vi "深国电程序控制old.vi"(11 "槽位号":i16) -> ()   [LabVIEW 2012]
doc: "打开板卡操作，输出板卡句柄！当有多个板卡时，根据板卡索引号打开不同板卡！\n如果同时使用一块板卡的多种功能，可将输出句柄连接到不同的功能任务中。\n此VI是创建所有任务的前提！"
uses:
  P3060.dll
panel:
  out "波形图":i32[](graph)
  in  "read":bool caption="确定按钮"
  in  "LED¿ØÖÆû":bool
  in  "FPGA-Bit文件路径":path
  in  "加载程序":bool caption="确定按钮"
  in  "取消按钮":bool
  out "error out":errorcluster caption="错误输出"
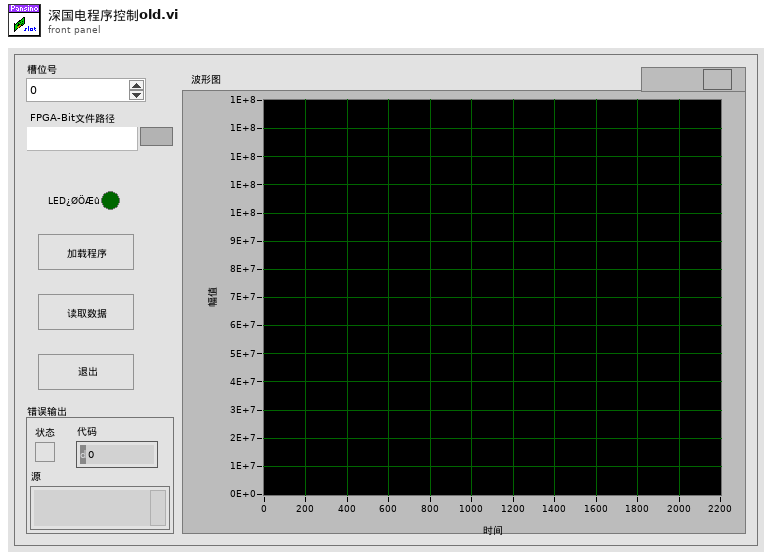
[diagram p1: front panel]
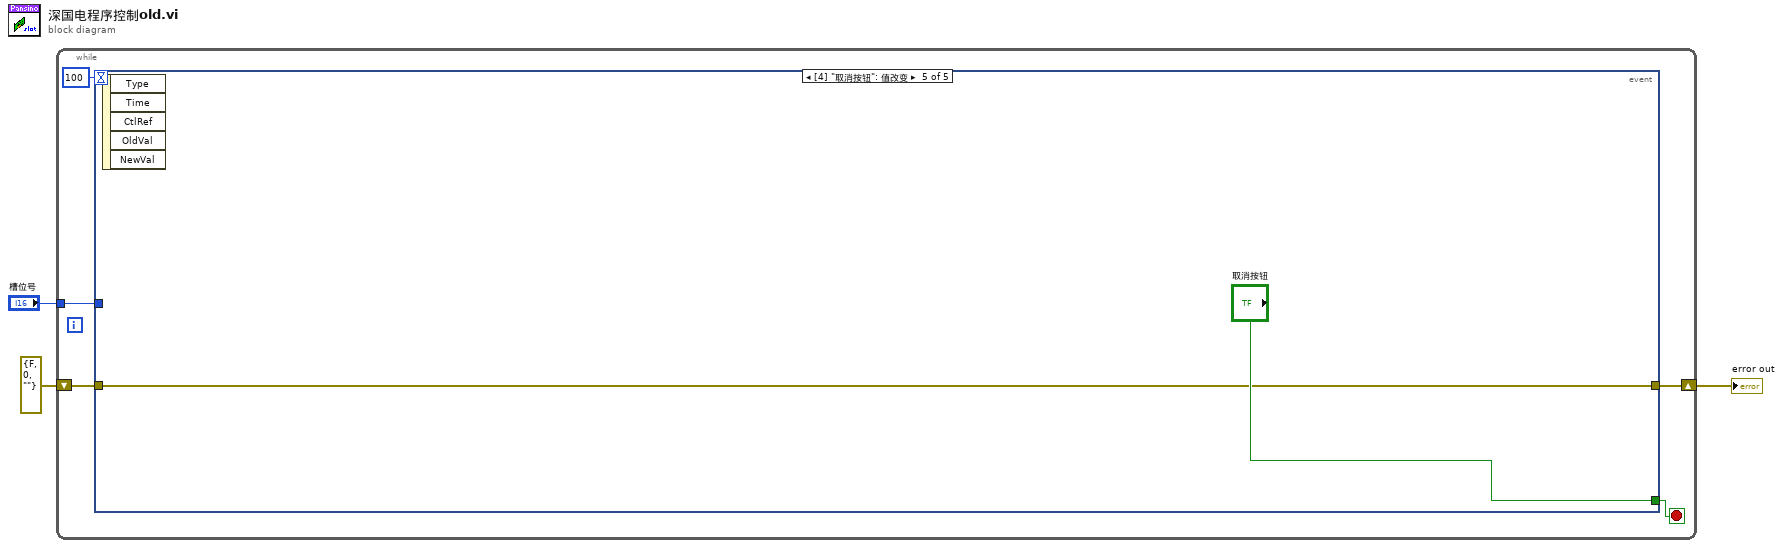
[diagram p0: block diagram]
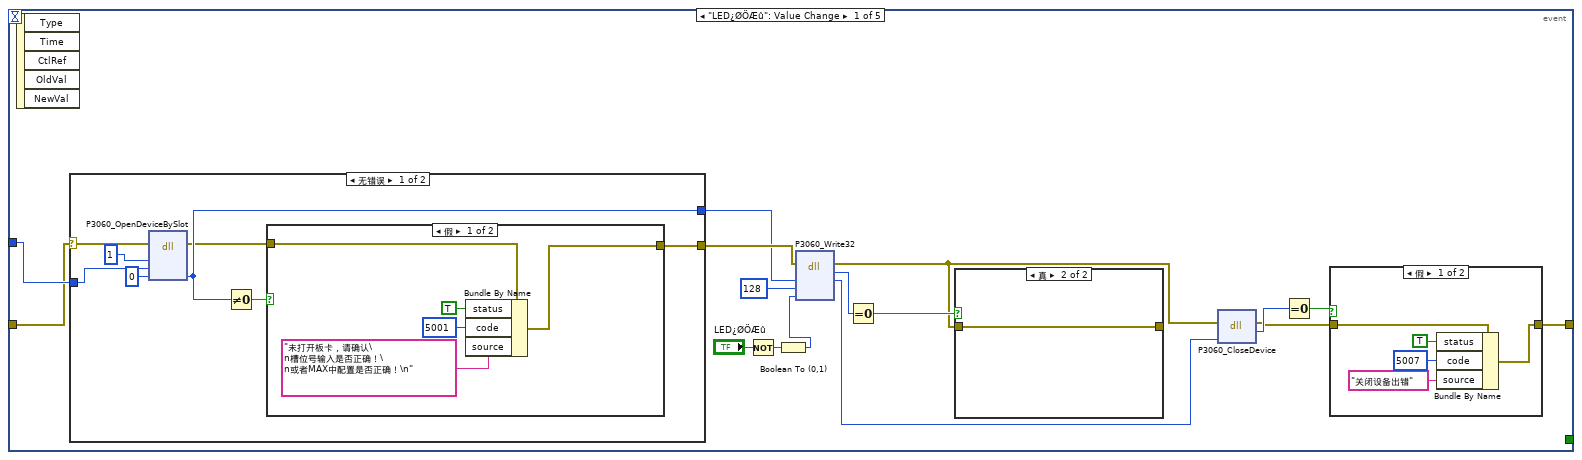
[diagram p2: hidden frame]
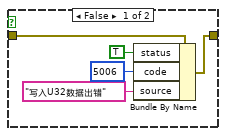
[diagram p3: hidden frame]
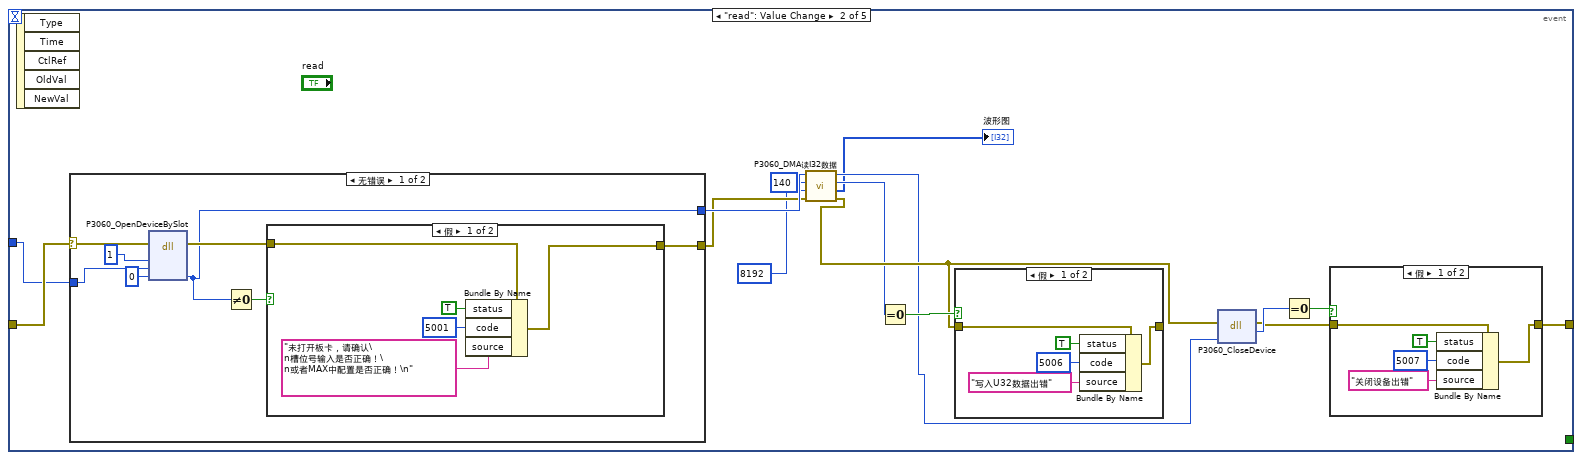
[diagram p7: hidden frame]
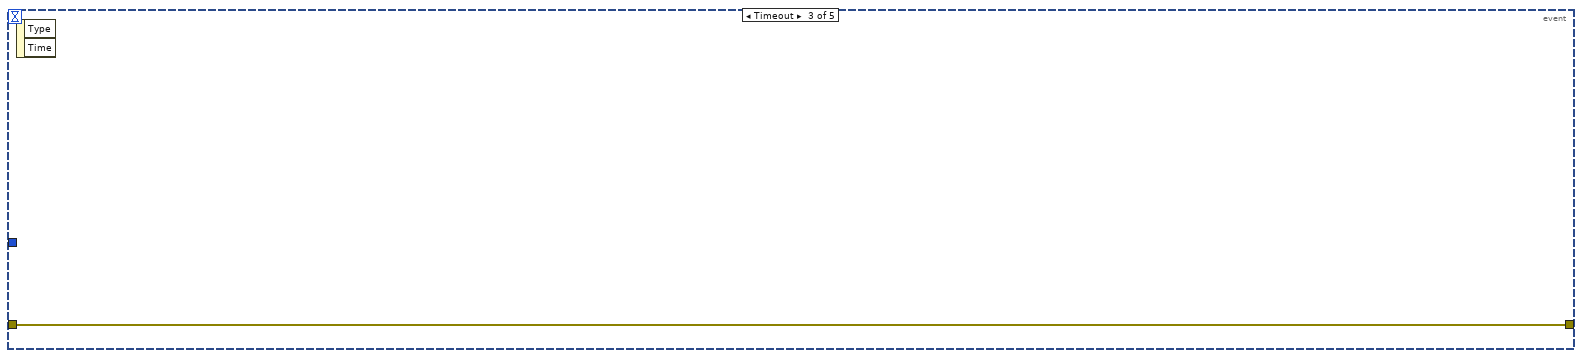
[diagram p12: hidden frame]
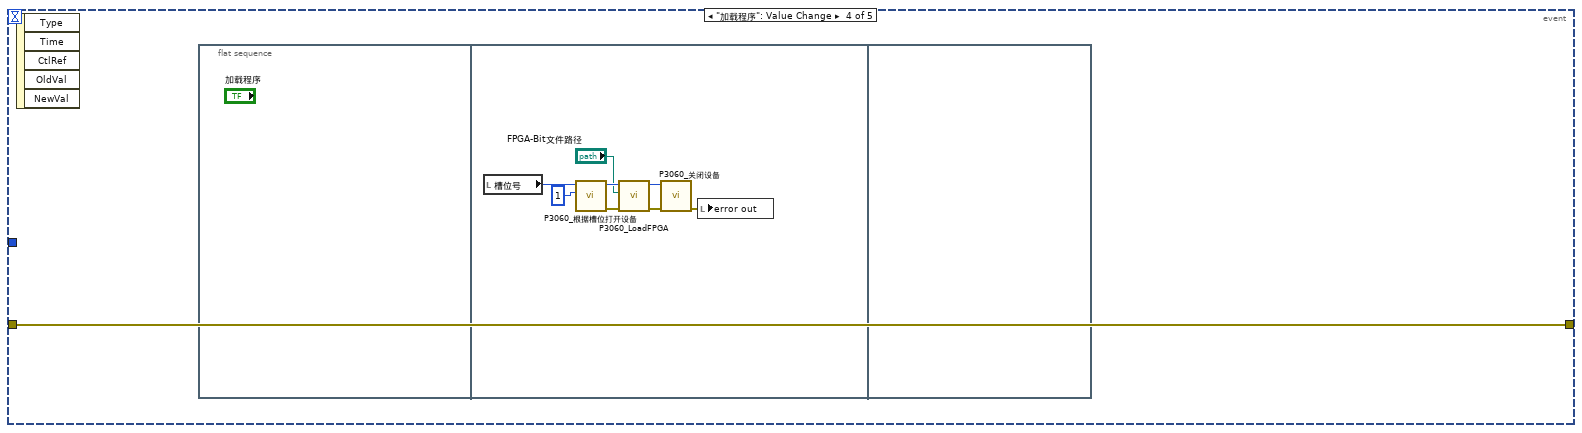
[diagram p13: hidden frame]
diagram:
  n1 = while {
    tunnel: "槽位号" -> [w8]
    shift-right: [w7] -> w1
    shift-left: errorcluster {"status"=FALSE, "code"=0, "source"=""} ("error IO") -> [w6]
    stop <- w4 stop-if-true
    n2 = event shown="[4] \"取消按钮\": 值改变" {
      selector: _ -> [_ _ _ _ _]
      dyn-events: _ -> [_ _ _ _ _]
      timeout: 100 -> [_ _ _ _ _]
      tunnel: [_ _ _ _ "取消按钮"] -> w4
      tunnel: w8 -> [w14 w52 _ _ _]
      tunnel: [w12 w62 w94 w95 w104] -> w7
      tunnel: w6 -> [w13 w61 w94 w95 w104]
      event "LED¿ØÖÆû": Value Change {
        n3 = event-data() -> ()  [unwired: 1 in, 5 out]
        n4 = case shown="无错误" w13 {
          selector: w13 -> [w44 w51]
          tunnel: [w41 w51] -> w19
          tunnel: w14 -> [w43 _]
          tunnel: [w40 _] -> w17
          frame No Error {
            n5 = dll-call lib="P3060.dll" fn="P3060_OpenDeviceBySlot"(error in=w44, "Classis"=i16 1, "槽位号"=w43, "设备句柄"=0) -> (error out=w37:errorcluster, "设备句柄"=w40:i32)  [unwired: 5 in, 1 out]
            n6 = Not Equal To 0?(x=w40) -> (x != 0?=w42:bool)
            n7 = case shown="假" w42 {
              tunnel: w37 -> [w49 w50]
              tunnel: [w45 w50] -> w41
              frame False {
                n8 = Bundle By Name(cluster=w49, "status"=TRUE, "code"=5001, "source"="未打开板卡，请确认\n槽位号输入是否正确！\n或者MAX中配置是否正确！\n") -> (w45:errorcluster)
              }
              frame True {
              }
            }
          }
          frame Error {
          }
        }
        n9 = Not(x="LED¿ØÖÆû") -> (.not. x?=w10:bool)
        n10 = Boolean To (0,1)(Boolean=w10) -> (0, 1=w11:i16)
        n11 = dll-call lib="P3060.dll" fn="P3060_Write32"(error in=w19, "hDev"=w17, "Offset"=u32 128, "data"=w11) -> (error out=w18:errorcluster, "return"=w21:i32, "hDev"=w16:i32)  [unwired: 4 in, 1 out]
        n12 = Equal To 0?(x=w21) -> (x = 0?=w20:bool)
        n13 = case shown="真" w20 {
          tunnel: [w28 w30] -> _
          tunnel: w18 -> [w29 w30]
          frame False {
            n14 = Bundle By Name(cluster=w29, "status"=TRUE, "code"=5006, "source"="写入U32数据出错") -> (w28:errorcluster)
          }
          frame True {
          }
        }
        n15 = dll-call lib="P3060.dll" fn="P3060_CloseDevice"(error in=w18, "hDev"=w16) -> (error out=w22:errorcluster, "hDevOut"=w24:i32)  [unwired: 3 in, 1 out]
        n16 = Equal To 0?(x=w24) -> (x = 0?=w23:bool)
        n17 = case shown="假" w23 {
          tunnel: [w34 w36] -> w12
          tunnel: w22 -> [w35 w36]
          frame False {
            n18 = Bundle By Name(cluster=w35, "status"=TRUE, "code"=5007, "source"="关闭设备出错") -> (w34:errorcluster)
          }
          frame True {
          }
        }
      }
      event "read": Value Change {
        n19 = event-data() -> ()  [unwired: 1 in, 5 out]
        n20 = case shown="无错误" w61 {
          selector: w61 -> [w86 w93]
          tunnel: [w82 w93] -> w59
          tunnel: w52 -> [w85 _]
          tunnel: [w79 _] -> w60
          frame No Error {
            n21 = dll-call lib="P3060.dll" fn="P3060_OpenDeviceBySlot"(error in=w86, "Classis"=i16 1, "槽位号"=w85, "设备句柄"=0) -> (error out=w83:errorcluster, "设备句柄"=w79:i32)  [unwired: 5 in, 1 out]
            n22 = Not Equal To 0?(x=w79) -> (x != 0?=w84:bool)
            n23 = case shown="假" w84 {
              tunnel: w83 -> [w91 w92]
              tunnel: [w87 w92] -> w82
              frame False {
                n24 = Bundle By Name(cluster=w91, "status"=TRUE, "code"=5001, "source"="未打开板卡，请确认\n槽位号输入是否正确！\n或者MAX中配置是否正确！\n") -> (w87:errorcluster)
              }
              frame True {
              }
            }
          }
          frame Error {
          }
        }
        n25 = call "P3060_DMA读I32数据.vi"("错误输入"=w59, "数据长度"=u32 8192, "偏移地址"=u32 140, "句柄输入"=w60) -> ("错误输出"=w58:errorcluster, "读I32数据"=→"波形图":i32[], "返回值"=w57:i32, "句柄输出"=w56:i32)  [unwired: 4 in]
        n26 = Equal To 0?(x=w57) -> (x = 0?=w63:bool)
        n27 = case shown="假" w63 {
          tunnel: [w70 w72] -> _
          tunnel: w58 -> [w71 w72]
          frame False {
            n28 = Bundle By Name(cluster=w71, "status"=TRUE, "code"=5006, "source"="写入U32数据出错") -> (w70:errorcluster)
          }
          frame True {
          }
        }
        n29 = dll-call lib="P3060.dll" fn="P3060_CloseDevice"(error in=w58, "hDev"=w56) -> (error out=w64:errorcluster, "hDevOut"=w66:i32)  [unwired: 3 in, 1 out]
        n30 = Equal To 0?(x=w66) -> (x = 0?=w65:bool)
        n31 = case shown="假" w65 {
          tunnel: [w76 w78] -> w62
          tunnel: w64 -> [w77 w78]
          frame False {
            n32 = Bundle By Name(cluster=w77, "status"=TRUE, "code"=5007, "source"="关闭设备出错") -> (w76:errorcluster)
          }
          frame True {
          }
        }
      }
      event Timeout {
        n33 = event-data() -> ()  [unwired: 1 in, 2 out]
      }
      event "加载程序": Value Change {
        n34 = event-data() -> ()  [unwired: 1 in, 5 out]
        n35 = flat-sequence {
          frame #0 {
          }
          frame #1 {
            n36 = local read "槽位号"() -> (w103:i16)
            n37 = call "P3060_根据槽位打开设备.vi"("机箱号"=i16 1, "槽位号"=w103) -> ("error out"=w99:errorcluster, "句柄输出"=w97:i32)  [unwired: 8 in]
            n38 = call "P3060_LoadFPGA.vi"("错误输入"=w99, "Bit文件路径"="FPGA-Bit文件路径", "句柄输入"=w97) -> ("错误输出"=w101:errorcluster, "句柄输出"=w100:i32)  [unwired: 6 in, 1 out]
            n39 = call "P3060_关闭设备.vi"("error in (no error)"=w101, "句柄输入"=w100) -> ("error out"=w102:errorcluster)  [unwired: 9 in]
            n40 = local write "error out"(w102) -> ()
          }
          frame #2 {
          }
        }
      }
      event "取消按钮": Value Change {
        n41 = event-data() -> ()  [unwired: 1 in, 5 out]
      }
    }
  }
  "error out" <- w1
